vi "ServosTesten.vi"() -> ()   [LabVIEW 2010]
uses:
  <vilib>/rvi/interface/nirviOpenFPGA/nirviOpenFPGA.xnode
  C:/Users/HAGAR-IV/Desktop/Zeugs/Johnny/pertrasgc fpga/FPGA-Programm-10-14.vi
  <vilib>/userDefined/High Color/nirio_resource_hc.ctl
  <vilib>/rvi/interface/nirviReadWriteControl/nirviReadWriteControl.xnode
  <vilib>/rvi/errors/niLvFpgaWhatHappensToTopLevelVI.ctl
  <vilib>/rvi/interface/common/niFpgaNodeNameForErrorReporting.ctl
  <vilib>/rvi/errors/niLvFpgaAdjustHostInterfaceError.vi
  <vilib>/rvi/interface/nirviMethod/nirviMethod.xnode
  <vilib>/rvi/interface/nirviCloseFPGA/nirviCloseFPGA.xnode
  C:/Users/HAGAR-IV/Desktop/Zeugs/markus/version feb 2012/FPGA Bitfiles/pertrasgcfpga2_FPGATarget_FPGA-Programm-10_6A1F8A79.lvbitx
  NiFpgaLv.dll
  <vilib>/Utility/error.llb/Error Cluster From Error Code.vi
  <vilib>/FPGAPlugInAG/cRIO-9114/niLvFpga_Close_cRIO-9114.vi
panel:
  in  "stop":bool
  in  "ServosWarmHigh (us)KaltHigh(us)":T1
  in  "ServoTrap2kalt":bool
  in  "ServoTrap1kalt":bool
  in  "ServosPeriode(us)":u32=10
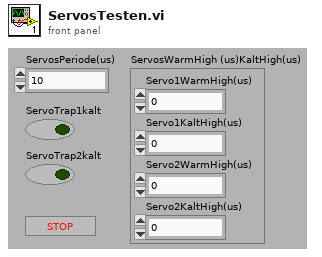
[diagram p1: front panel]
types:
  T1 = cluster{"Servo1WarmHigh(us)":u32, "Servo1KaltHigh(us)":u32, "Servo2WarmHigh(us)":u32, "Servo2KaltHigh(us)":u32}
  T2 = cluster{"MainCol1-2":bool, "Valve1-2":bool, "Spare1-2":bool, "Spare1-1":bool, "Valve1-1":bool, "MainCol1-1":bool, "Drier":bool, "Licor":bool, "ECD2":bool, "Oven2":bool, "Spare2-1":bool, "Col2-2":bool, "Col2-1":bool, "ECD1":bool}
  T3 = typedef "niFpgaNodeNameForErrorReporting.ctl" = enum16{"Open FPGA VI Reference", "Read/Write Control", "Invoke Method: Abort", "Invoke Method: Acknowledge IRQ", "Invoke Method: Download", "Invoke Method: FIFO.Configure", "Invoke Method: FIFO.Read", "Invoke Method: FIFO.Start", "Invoke Method: FIFO.Stop", "Invoke Method: FIFO.Write", "Invoke Method: Reset", "Invoke Method: Run", "Invoke Method: Wait on IRQ", "Close FPGA VI Reference"}
  T4 = typedef "niLvFpgaWhatHappensToTopLevelVI.ctl" = enum16{"top level VI scripted behind XNode", "top level VI inlined behind XNode"}
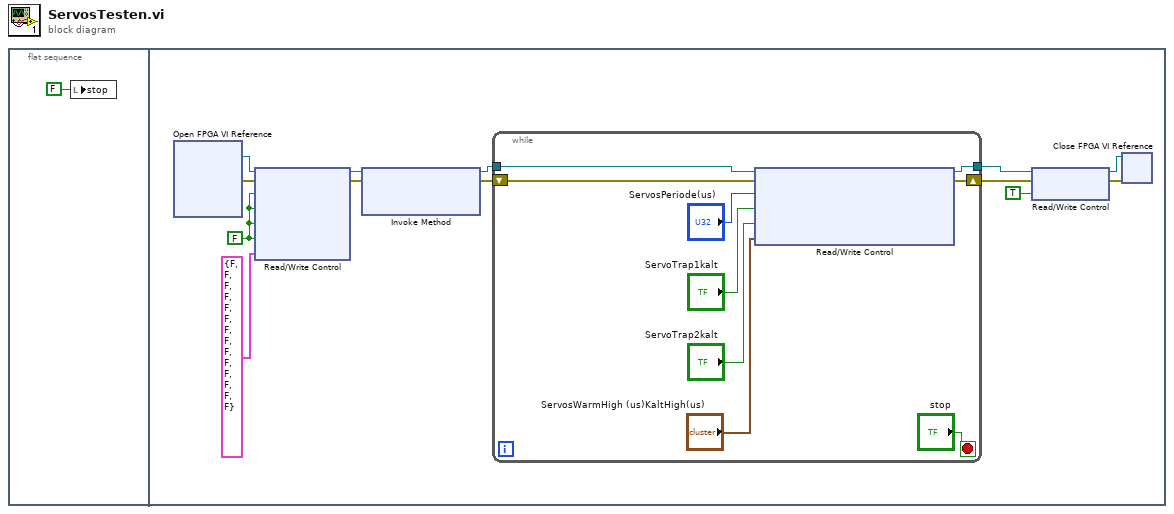
[diagram p0: block diagram]
diagram:
  n1 = flat-sequence {
    frame #0 {
      n2 = local write "stop"(FALSE ("stop")) -> ()
    }
    frame #1 {
      w13 = FALSE ("Heizen?Trap1")
      n3 = xnode "Open FPGA VI Reference"() -> ("FPGA VI Reference Out"=w14:refnum<k20>, "error out"=w10:errorcluster)  [unwired: 2 in]
      n4 = xnode "Read/Write Control"("FPGA VI Reference In"=w14, "error in"=w10, "Heizen?Trap1"=w13, "Heizen?Trap2"=w13, "Heizen?Mach1"=w13, "Heizen?Mach2"=w13, "LHHeizen?"=T2 {"MainCol1-2"=FALSE, "Valve1-2"=FALSE, "Spare1-2"=FALSE, "Spare1-1"=FALSE, "Valve1-1"=FALSE, "MainCol1-1"=FALSE, "Drier"=FALSE, "Licor"=FALSE, "ECD2"=FALSE, "Oven2"=FALSE, "Spare2-1"=FALSE, "Col2-2"=FALSE, "Col2-1"=FALSE, "ECD1"=FALSE}) -> ("FPGA VI Reference Out"=w11:refnum<k20>, "error out"=w9:errorcluster)
      n5 = xnode "Invoke Method"("FPGA VI Reference In"=w11, "error in"=w9) -> ("FPGA VI Reference Out"=w8:refnum<k20>, "error out"=w7:errorcluster)  [unwired: 1 in]
      n6 = while {
        tunnel: w8 -> [w147]
        shift-right: [w145] -> w5
        shift-left: w7 -> [w146]
        tunnel: [w144] -> w6
        stop <- "stop" stop-if-true
        n7 = xnode "Read/Write Control"("FPGA VI Reference In"=w147, "error in"=w146, "ServosPeriode(us)"="ServosPeriode(us)", "ServoTrap1kalt"="ServoTrap1kalt", "ServoTrap2kalt"="ServoTrap2kalt", "ServosWarmHigh (us)KaltHigh(us)"="ServosWarmHigh (us)KaltHigh(us)") -> ("FPGA VI Reference Out"=w144:refnum<k20>, "error out"=w145:errorcluster)
      }
      n8 = xnode "Read/Write Control"("FPGA VI Reference In"=w6, "error in"=w5, "global stop"=TRUE) -> ("FPGA VI Reference Out"=w3:refnum<k20>, "error out"=w2:errorcluster)
      n9 = xnode "Close FPGA VI Reference"("FPGA VI Reference In"=w3, "error in"=w2) -> ()  [unwired: 1 out]
    }
  }
